vi "GoToBallPlacementPositionTactic.vi"(7 "firstCall":bool, 8 "error in (no error)":errorcluster, 9 "Game in":refnum<class "Game.lvclass">, 10 "Robot":refnum<class "Robot.lvclass">, 11 "GoToBallPlacementPositionTactic in":refnum<class "GoToBallPlacementPositionTactic.lvclass">) -> (0 "error out":errorcluster, 2 "Robot out":refnum<class "Robot.lvclass">, 3 "GoToBallPlacementPositionTactic out":refnum<class "GoToBallPlacementPositionTactic.lvclass">)   [LabVIEW 2021, in "GoToBallPlacementPositionTactic.lvclass"]
uses:
  GoToBallPlacementPositionTactic.lvclass
  D:/RoboIme/horie/SSL_AI/Tactic_class/Tactic.lvclass
  Robot_class/Robot.lvclass
  Game_class/Game.lvclass
  Robot_class/tactics.ctl
  StatesGoToBallPlacementPositionTactic.ctl
  Tactic_class/Tactic.lvclass/Tactic.ctl
  Skillbook_class/Skillbook.lvclass/Skillbook.ctl
  Robot_class/Robot.lvclass/Robot.ctl
  GoToBallPlacementPositionTactic.lvclass/GoToBallPlacementPositionTactic.ctl
  Skillbook_class/Read GoToBallPlacementPositionSkill.vi
  Tactic_class/Read Skillbook.vi
  Write States.vi
  Robot_class/Write tactic.vi
  Skillbook_class/Skillbook.lvclass
  GoToBallPlacementPositionSkill_class/GoToBallPlacementPositionSkill.lvclass
panel:
  out "x .or. y?":bool
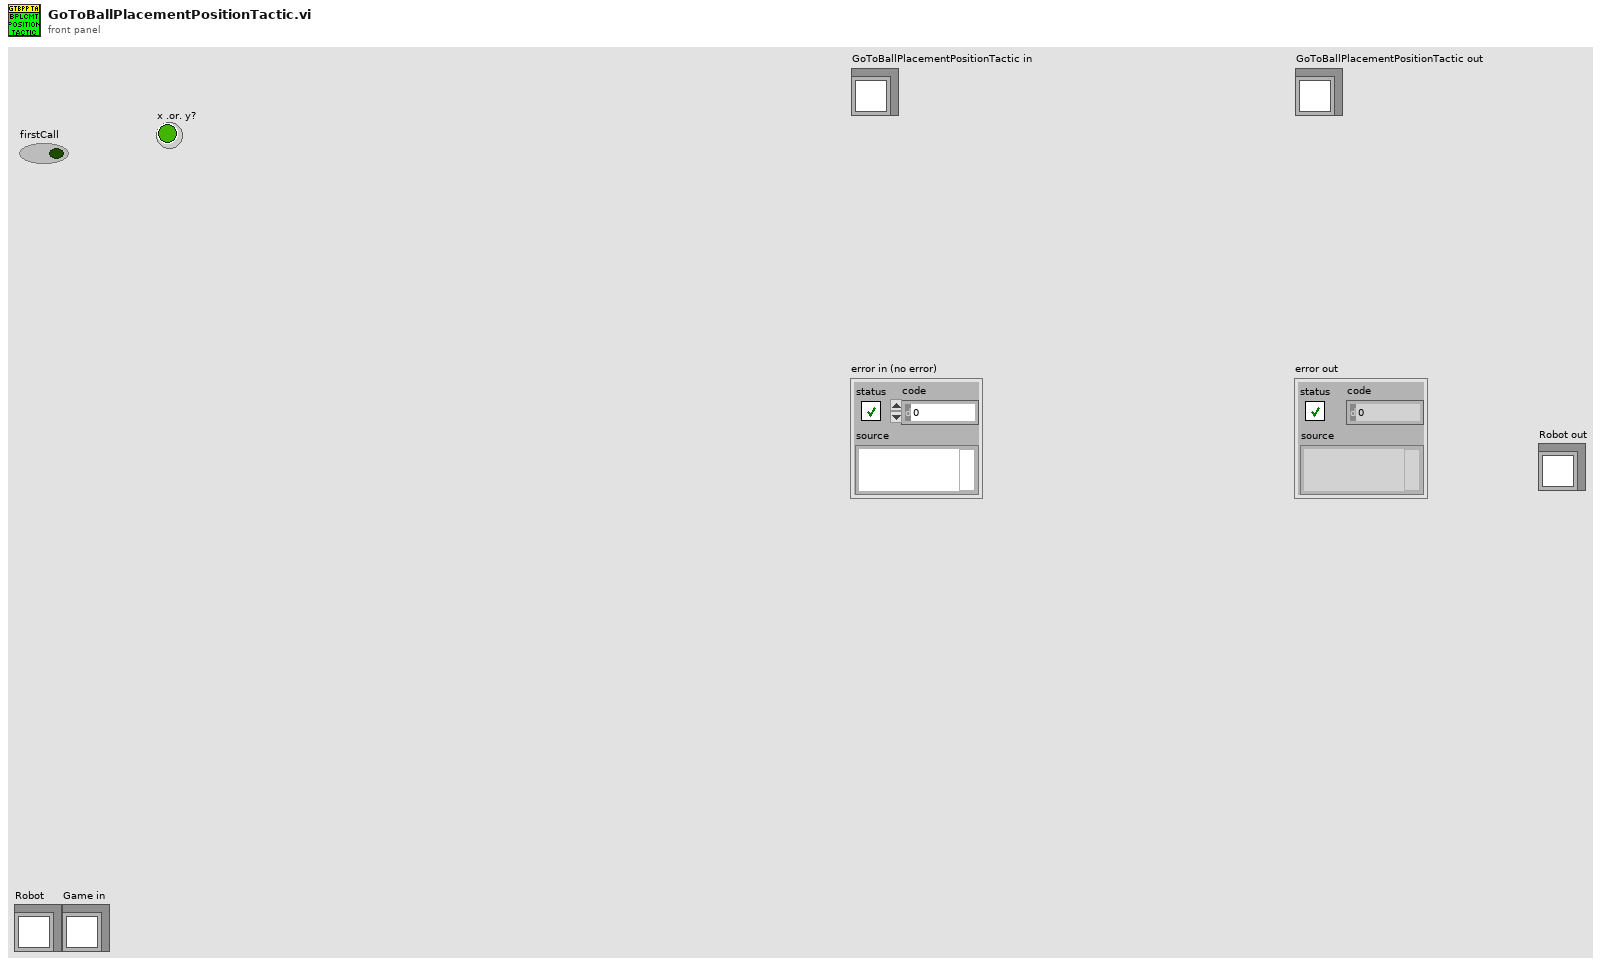
[diagram p1: front panel]
types:
  T1 = typedef "GoToBallPlacementPositionTactic.lvclass/StatesGoToBallPlacementPositionTactic.ctl" = enum16{"GoToPosition", "Exit"}
  T2 = typedef "tactics.ctl" = enum16{"GoToBallPlacementPosition", "PlaceBall", "GoToBallPlacement", "5Robots", "BallPlacementEnemy", "ReceivePassInFuturePoint", "Roller", "PrepareRollToPassRollerGoTo", "PrepareRollToPassReceiverGoTo", "WaitRoll", "PositionToRoll", "PenaltyAttacker", "PassObserver", "PenaltyDefense", "TableReceiverTactic", "Test", "DefendGoal", "Marker", "FollowAttacker", "DefendArea", "Shoot", "AttackerAimGoal", "AttackerBallOutOfField", "AttackerBlock", "AttackerStop", "Duelist", "Halt", "ZigZag", "GoTo", "Timeout", "KickToBestRobot", "KickToPassReceiver", "PositionToReceivePass", "WaitPass"}
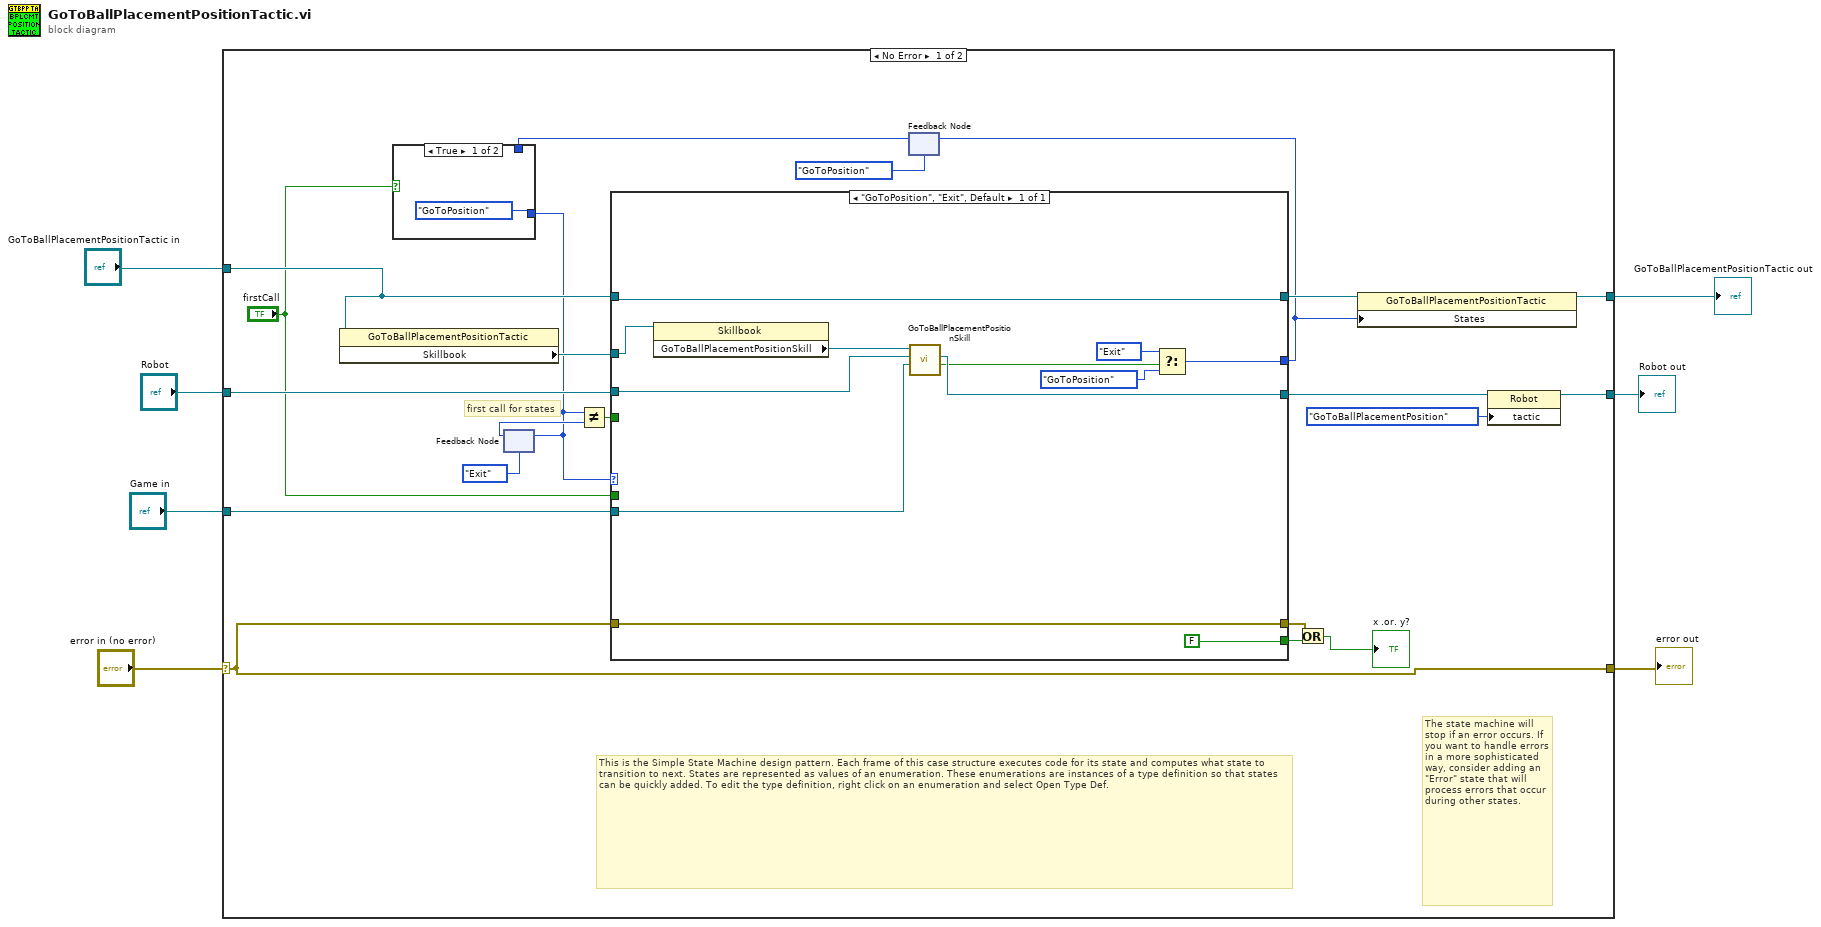
[diagram p0: block diagram]
diagram:
  n1 = case shown="No Error" "error in (no error)" {
    selector: "error in (no error)" -> [w21 w44]
    tunnel: [w21 w44] -> w3
    tunnel: [w20 w43] -> w1
    tunnel: "GoToBallPlacementPositionTactic in" -> [w22 w43]
    tunnel: [w19 _] -> w7
    tunnel: "Robot" -> [w17 _]
    tunnel: "Game in" -> [w16 _]
    frame No Error {
      # "first call for states"
      # "The state machine will stop if an error occurs. If you want to handle errors in a more sophisticated way, consider adding an \"Error\" state that will process errors that occur during other states."
      # "This is the Simple State Machine design pattern. Each frame of this case structure executes code for its state and computes what state to transition to next. States are represented as values of an enumeration. These enumerations are instances of a type definition so that states can be quickly added. To edit the type definition, right click on an enumeration and select Open Type Def."
      n2 = property class="GoToBallPlacementPositionTactic"(reference=w22) -> ("Skillbook"=w25:refnum<class "Skillbook.lvclass">)  [unwired: 1 in, 2 out]
      n3 = feedback #1(StatesGoToBallPlacementPositionTactic."Exit" ("States")) -> (w13:T1)
      n4 = feedback #2(StatesGoToBallPlacementPositionTactic."GoToPosition" ("States")) -> (w15:T1)
      n5 = case shown="True" "firstCall" {
        tunnel: [StatesGoToBallPlacementPositionTactic."GoToPosition" ("States") w30] -> w12
        tunnel: w15 -> [_ w30]
        frame True {
        }
        frame False {
        }
      }
      n6 = feedback-in #1(w12) -> ()
      n7 = Not Equal?(x=w12, y=w13) -> (x != y?=w11:bool)
      n8 = case shown="\"GoToPosition\", \"Exit\", Default" w12 {
        tunnel: [FALSE ("Stop Loop?")] -> w27
        tunnel: w25 -> [w41]
        tunnel: w17 -> [w36]
        tunnel: [w37] -> w23
        tunnel: [w42] -> w24
        tunnel: w22 -> [w42]
        tunnel: w16 -> [w35]
        tunnel: [w40] -> w28
        tunnel: w21 -> [w40]
        tunnel: [w32] -> w8
        tunnel: "firstCall" -> [_]
        tunnel: w11 -> [_]
        frame "GoToPosition", "Exit", Default {
          n9 = property class="Skillbook"(reference=w41) -> ("GoToBallPlacementPositionSkill"=w38:refnum<class "GoToBallPlacementPositionSkill.lvclass">)  [unwired: 1 in, 2 out]
          n10 = call "GoToBallPlacementPositionSkill.vi"("Game"=w35, "Robot"=w36, "GoToBallPlacementPositionSkill in"=w38) -> ("robotPositionedToReceiveBall"=w34:bool, "Robot out"=w37:refnum<class "Robot.lvclass">)  [unwired: 5 in, 2 out]
          n11 = Select(t=StatesGoToBallPlacementPositionTactic."Exit", s=w34, f=StatesGoToBallPlacementPositionTactic."GoToPosition" ("States")) -> (s? t:f=w32:T1)
        }
      }
      n12 = feedback-in #2(w8) -> ()
      n13 = Or(x=w28, y=w27) -> (x .or. y?=→"x .or. y?":bool)
      n14 = property class="GoToBallPlacementPositionTactic"(reference=w24, "States"=w8) -> (reference out=w20:refnum<class "GoToBallPlacementPositionTactic.lvclass">)  [unwired: 1 in, 1 out]
      n15 = property class="Robot"(reference=w23, "tactic"=tactics."GoToBallPlacementPosition") -> (reference out=w19:refnum<class "Robot.lvclass">)  [unwired: 1 in, 1 out]
    }
    frame Error {
    }
  }
  "error out" <- w3
  "GoToBallPlacementPositionTactic out" <- w1
  "Robot out" <- w7
